vi "VCS Get Position Marker Parameter.vi"(6 "error in (no error)":errorcluster, 9 "axis in":cluster{"keyHandle":u32, "nodeId":u16}={"keyHandle"=0, "nodeId"=1}) -> (0 "error out":errorcluster, 1 "position marker parameter":T1 {"positionMarkerMode" items=["continuous", "single", "multiple"]; "positionMarkerEdgeType" items=["both edges", "rising edge", "falling edge"]}, 3 "axis out":cluster{"keyHandle":u32, "nodeId":u16}={"keyHandle"=0, "nodeId"=1})   [LabVIEW 2010]
doc: "<B>VCS_GetPositionMarkerParameter</B> reads all parameters for position marker method."
uses:
  Resources/EposCmd.dll
  Resources/EposCmd64.dll
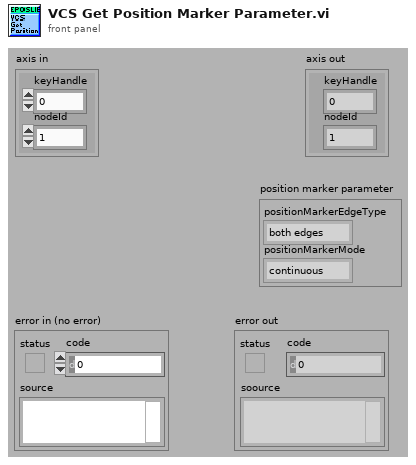
[diagram p1: front panel]
types:
  T1 = cluster{"positionMarkerEdgeType":u8, "positionMarkerMode":u8}
  T2 = cluster{"pPositionMarkerEdgeType":u8, "pPositionMarkerMode":u8}
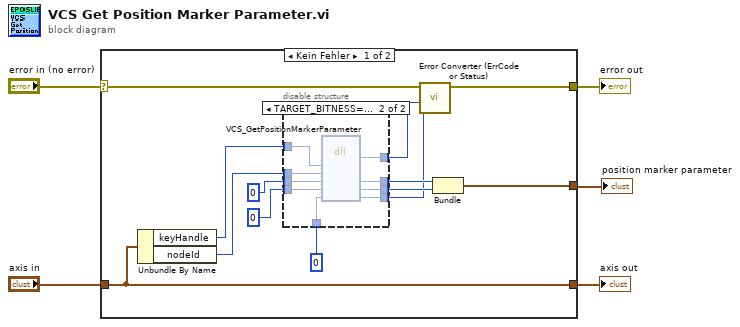
[diagram p0: block diagram]
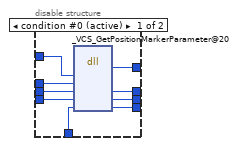
[diagram p2: hidden frame]
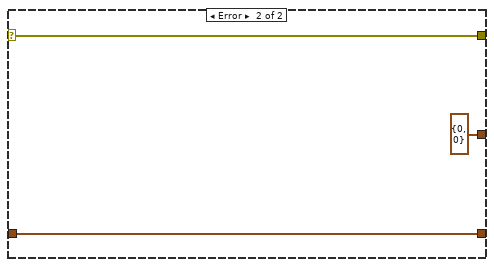
[diagram p3: hidden frame]
diagram:
  n1 = case shown="Kein Fehler" "error in (no error)" {
    selector: "error in (no error)" -> [w16 w38]
    tunnel: "axis in" -> [w18 w39]
    tunnel: [w18 w39] -> w4
    tunnel: [w17 w38] -> w3
    tunnel: [w10 T2 {"pPositionMarkerEdgeType"=0, "pPositionMarkerMode"=0}] -> w1
    frame No Error {
      n2 = Unbundle By Name(w18) -> ("keyHandle"=w14:u32, "nodeId"=w13:u16)
      n3 = disable-structure shown="TARGET_BITNESS==64" {
        disable-tunnel: u32 0 ("pErrorCode") -> [w27 w36]
        disable-tunnel: w14 -> [w26 w35]
        disable-tunnel: w13 -> [w25 w34]
        disable-tunnel: [w24 w33] -> w12
        disable-tunnel: [w23 w32] -> w11
        disable-tunnel: u8 0 ("pPositionMarkerMode") -> [w22 w31]
        disable-tunnel: u8 0 ("pPositionMarkerEdgeType") -> [w21 w30]
        disable-tunnel: [w20 w29] -> w7
        disable-tunnel: [w19 w28] -> w6
        frame condition #0 (active) {
          n4 = dll-call lib="C:/Sources/LabView/maxon EPOS/Resources/EposCmd.*" fn="_VCS_GetPositionMarkerParameter@20"("KeyHandle"=w26, "NodeId"=w25, "pPositionMarkerEdgeType"=w21, "pPositionMarkerMode"=w22, "pErrorCode"=w27) -> ("Rückgabetyp"=w19:i32, "pPositionMarkerEdgeType"=w24:u8, "pPositionMarkerMode"=w23:u8, "pErrorCode"=w20:u32)  [unwired: 5 in, 2 out]
        }
        frame condition #1 {
          n5 = dll-call lib="C:/setup/Resources/EposCmd64.*" fn="VCS_GetPositionMarkerParameter" ("EposCmd.dll:_VCS_GetPositionMarkerParameter@20")("KeyHandle"=w35, "NodeId"=w34, "pPositionMarkerEdgeType"=w30, "pPositionMarkerMode"=w31, "pErrorCode"=w36) -> ("Rückgabetyp"=w28:i32, "pPositionMarkerEdgeType"=w33:u8, "pPositionMarkerMode"=w32:u8, "pErrorCode"=w29:u32)  [unwired: 5 in, 2 out]
        }
      }
      n6 = call "Error Converter (ErrCode or Status).vi"("error code"=w7, "return type"=w6, "error in (no error)"=w16) -> ("error out"=w17:errorcluster)  [unwired: 7 in]
      n7 = Bundle("pPositionMarkerEdgeType"=w12, "pPositionMarkerMode"=w11) -> (w10:T2)  [unwired: 1 in]
    }
    frame Error {
    }
  }
  "error out" <- w3
  "axis out" <- w4
  "position marker parameter" <- w1
